vi "Read.vi"(8 "error in (no error)":errorcluster, 11 "VISA resource name":refnum<visa-resource-name>) -> (0 "error out":errorcluster, 2 "Message Received":string, 3 "VISA resource name out":refnum<visa-resource-name>)   [LabVIEW 2018, in "LTB-1.lvlib" / "3150.lvlib"]
doc: "Responsible for reading the read buffer of the device and parse the retrieved message based on the mode of communication."
uses:
  3150.lvlib
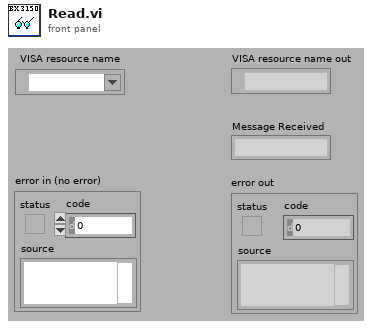
[diagram p1: front panel]
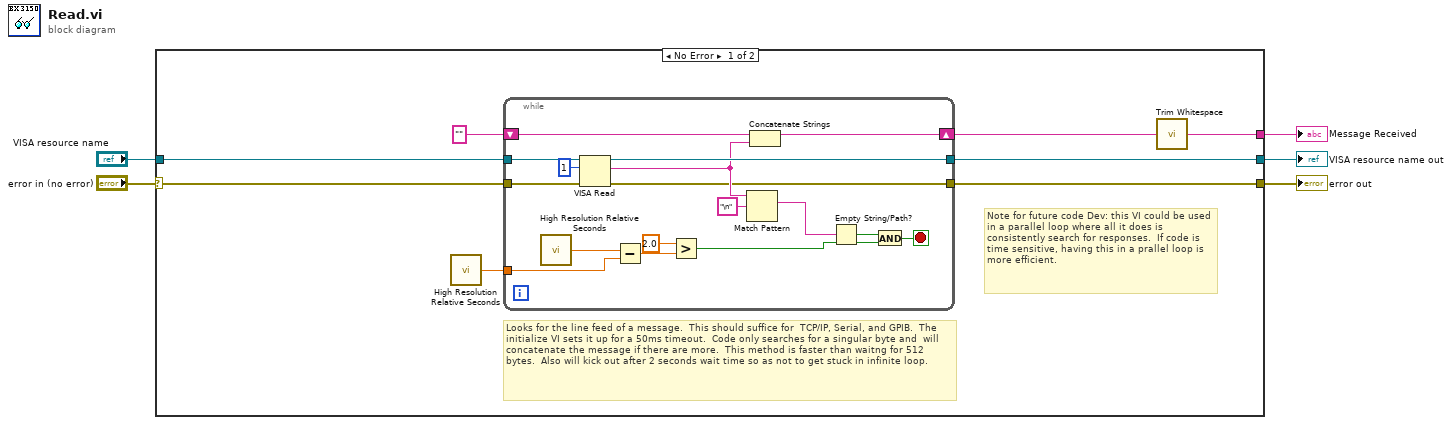
[diagram p0: block diagram]
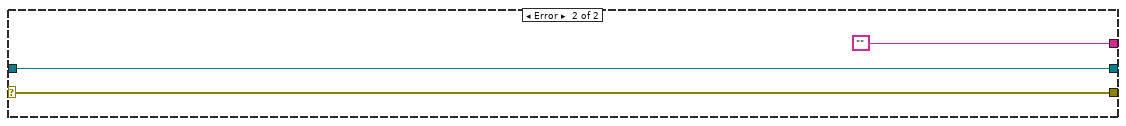
[diagram p2: hidden frame]
diagram:
  n1 = case shown="No Error" "error in (no error)" {
    selector: "error in (no error)" -> [w11 w33]
    tunnel: [w6 w33] -> w1
    tunnel: [w7 ""] -> w3
    tunnel: "VISA resource name" -> [w12 w31]
    tunnel: [w9 w31] -> w4
    frame No Error {
      # "Note for future code Dev: this VI could be used in a parallel loop where all it does is consistently search for responses.  If code is time sensitive, having this in a prallel loop is more efficient."
      # "Looks for the line feed of a message.  This should suffice for  TCP/IP, Serial, and GPIB.  The initialize VI sets it up for a 50ms timeout.  Code only searches for a singular byte and  will concatenate the message if there are more.  This method is faster than waitng for 512 bytes.  Also will kick out after 2 seconds wait time so as not to get stuck in infinite loop."
      n2 = call <vilib>:"High Resolution Relative Seconds.vi"() -> ("relative seconds"=w13:dbl)
      n3 = while {
        tunnel: w13 -> [w21]
        tunnel: w12 -> [w30]
        tunnel: w11 -> [w28]
        shift-right: [w27] -> w8
        shift-left: "" -> [w26]
        tunnel: [w25] -> w9
        tunnel: [w14] -> w6
        stop <- w15 stop-if-true
        n4 = call <vilib>:"High Resolution Relative Seconds.vi"() -> ("relative seconds"=w22:dbl)
        n5 = VISA Read(VISA resource name=w30, byte count=u32 1, error in (no error)=w28) -> (VISA resource name out=w25:refnum<visa-resource-name>, read buffer=w24:string, error out=w14:errorcluster)  [unwired: 1 out]
        n6 = Subtract(x=w22, y=w21) -> (x-y=w18:dbl)
        n7 = Greater?(x=2.0, y=w18) -> (0:w16:bool)
        n8 = Match Pattern(string=w24, regular expression="\n") -> (match substring=w20:string)  [unwired: 1 in, 3 out]
        n9 = Concatenate Strings(w26, w24) -> (w27:string)
        n10 = Empty String/Path?(string/path=w20) -> (empty?=w19:bool)
        n11 = And(x=w19, y=w16) -> (x .and. y?=w15:bool)
      }
      n12 = call <vilib>:"Trim Whitespace.vi"("string"=w8) -> ("trimmed string"=w7:string)  [unwired: 1 in]
    }
    frame Error {
    }
  }
  "VISA resource name out" <- w4
  "Message Received" <- w3
  "error out" <- w1
